vi "Reset.vi"   [LabVIEW 2018]
uses:
  <vilib>/Rock Robotics/WPI/ThirdParty/Sensors/navX/_TypeDefs/FRIC_navX_DeviceNumbersTypeDef.ctl
types:
  T1 = typedef "FRIC_navX_DeviceNumbersTypeDef.ctl" = enum16{"Dev0", "Dev1", "Dev2", "Dev3"}
  T2 = typedef "WPI_EncoderDevRef.ctl" = cluster{"DevStatus":errorcluster, "EncoderIndex":T3, "CounterIndex":T4, "DistancePerCount":dbl, "Decoding Type":T5}
  T3 = typedef "FPGA_EncoderIdx.ctl" = enum8{"Enc 0", "Enc 1", "Enc 2", "Enc 3", "Enc 4", "Enc 5", "Enc 6", "Enc 7", "Invalid"}
  T4 = typedef "FPGA_CounterCtrSystemIndex.ctl" = enum8{"Ctr 0", "Ctr 1", "Ctr 2", "Ctr 3", "Ctr 4", "Ctr 5", "Ctr 6", "Ctr 7", "Invalid"}
  T5 = typedef "WPI_EncoderType.ctl" = enum16{"1x", "2x", "4x"}
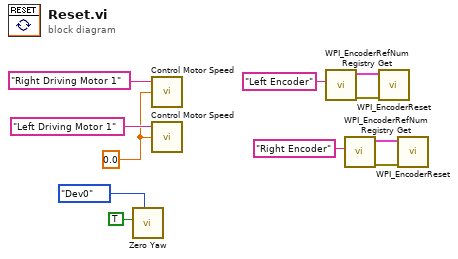
[diagram p0: block diagram]
diagram:
  w9 = 0.0 ("Speed")
  n1 = call <vilib>:"Zero Yaw.vi"("Device Number"=FRIC_navX_DeviceNumbersTypeDef."Dev0", "Zero"=TRUE) -> ()  [unwired: 10 in]
  n2 = call "Control Motor Speed.vi"("Speed"=w9, "Motor Name"="Right Driving Motor 1") -> ()  [unwired: 2 in]
  n3 = call "Control Motor Speed.vi"("Speed"=w9, "Motor Name"="Left Driving Motor 1") -> ()  [unwired: 2 in]
  n4 = call <vilib>:"WPI_EncoderRefNum Registry Get.vi"("refnum name"="Left Encoder") -> ("error out"=w6:errorcluster, "EncoderDevRef"=w5:T2)  [unwired: 9 in]
  n5 = call <vilib>:"WPI_EncoderRefNum Registry Get.vi"("refnum name"="Right Encoder") -> ("error out"=w3:errorcluster, "EncoderDevRef"=w2:T2)  [unwired: 9 in]
  n6 = call <vilib>:"WPI_EncoderReset.vi"("error in (no error)"=w6, "EncoderDevRef"=w5) -> ()  [unwired: 8 in, 2 out]
  n7 = call <vilib>:"WPI_EncoderReset.vi"("error in (no error)"=w3, "EncoderDevRef"=w2) -> ()  [unwired: 8 in, 2 out]
